vi "Create 256 Values Palette.vi"(5 "Image High Color":u32(colorbox), 7 "Image Low Color":u32(colorbox), 9 "Source Image Display Range":cluster{"Min Value":dbl, "Max Value":dbl}={"Min Value"=nan, "Max Value"=nan}, 10 "Interpolate?":bool, 11 "Palette Colors in":u32[](array[colorbox])) -> (0 "Color Scale Marker Values":T1(array[cluster]), 2 "1D U32 array":u32[](array[colorbox]), 3 "1D Color value array":cluster{"Red":u8, "Green":u8, "Blue":u8}[](array[cluster]))   [LabVIEW 2019]
uses:
  <vilib>/vision/NI_Vision_Development_Module.lvlib
panel:
  out "Color Ramp":dbl(ramp)
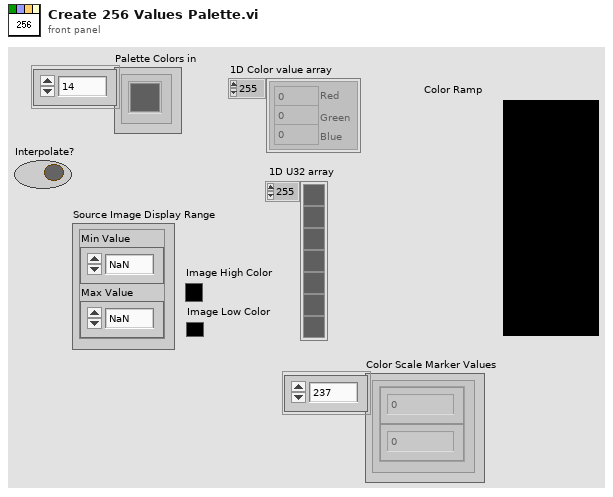
[diagram p1: front panel]
types:
  T1 = cluster{"Numeric Control":dbl, "Numeric Control":u32}[]
  T2 = typedef "For Loop Iteration Type.ctl" = enum16{"default", "first", "last", "out of range"}
  T3 = cluster{"Red (or Hue) value":u8, "Green (or Sat) value":u8, "Blue (or Light or Val) value":u8}[]
  T4 = cluster{"Red (or Hue) value":u8, "Green (or Sat) value":u8, "Blue (or Light or Val) value":u8}
  T5 = cluster{"Numeric Control":dbl, "Numeric Control":u32}
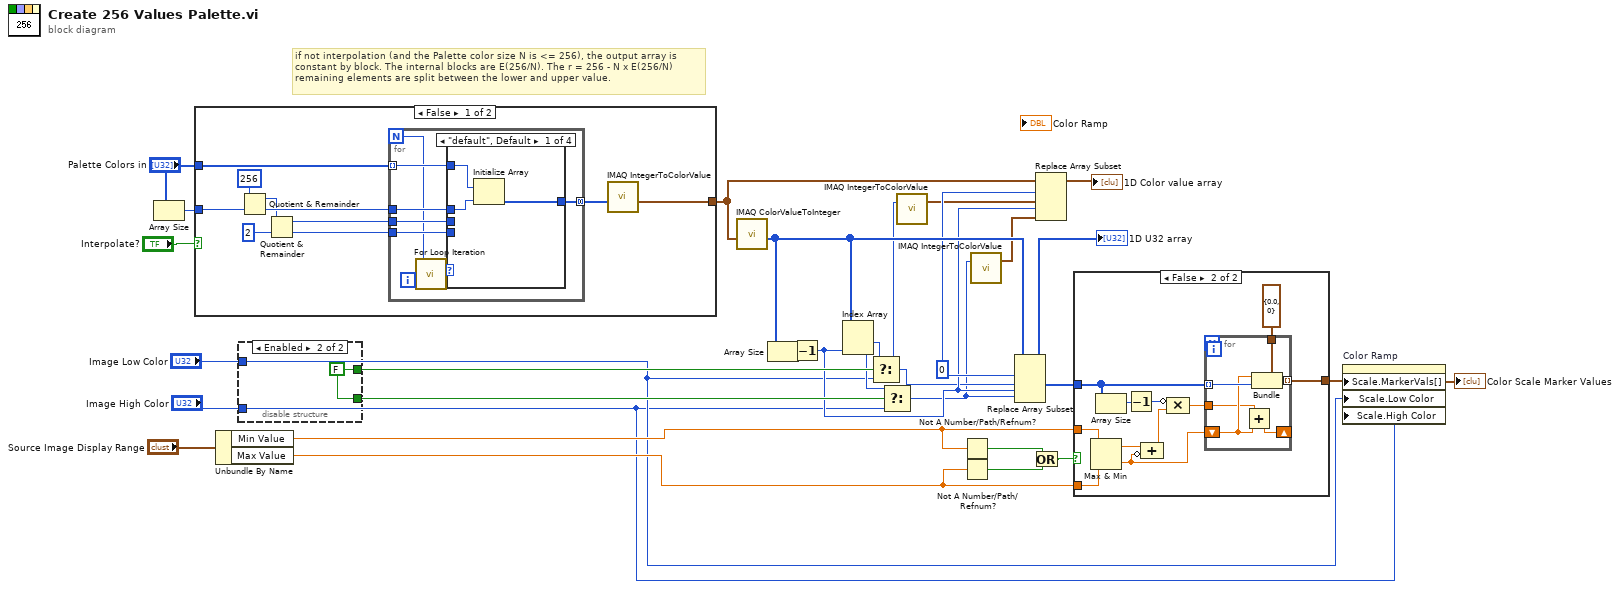
[diagram p0: block diagram]
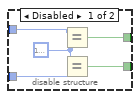
[diagram p2: hidden frame]
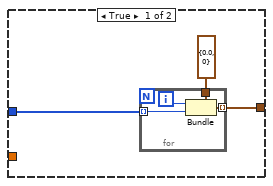
[diagram p3: hidden frame]
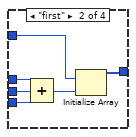
[diagram p4: hidden frame]
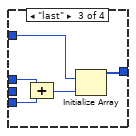
[diagram p5: hidden frame]
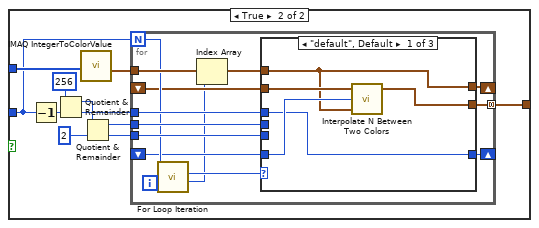
[diagram p7: hidden frame]
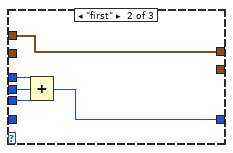
[diagram p8: hidden frame]
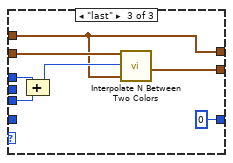
[diagram p9: hidden frame]
diagram:
  w9 = 0 ("index")
  # "if not interpolation (and the Palette color size N is <= 256), the output array is\nconstant by block. The internal blocks are E(256/N). The r = 256 - N x E(256/N)\nremaining elements are split between the lower and upper value."
  n1 = Array Size(array="Palette Colors in") -> (size(s)=w26:i32)
  n2 = case shown="False" "Interpolate?" {
    tunnel: w26 -> [w37 w61]
    tunnel: "Palette Colors in" -> [w32 w64]
    tunnel: [w28 w62] -> w10
    frame False {
      n3 = Quotient & Remainder(x=256, y=w37) -> (x-y*floor(x/y)=w35:i32, floor(x/y)=w36:i32)
      n4 = Quotient & Remainder(x=w35, y=2) -> (x-y*floor(x/y)=w33:i32, floor(x/y)=w31:i32)
      n5 = for {
        N -> [w38]
        tunnel: w36 -> [w43]
        tunnel: w31 -> [w45]
        tunnel: w33 -> [w44]
        tunnel: w32 -> [w41] mode=indexing
        tunnel: [w42] -> w29 mode=concatenating
        i -> [w40]
        n6 = call "For Loop Iteration.vi"("i"=w40, "N"=w38) -> ("Iteration"=w39:T2)  [unwired: 8 in, 1 out]
        n7 = case shown="\"default\", Default" w39 {
          tunnel: w45 -> [_ w54 w59 _]
          tunnel: w44 -> [_ w53 _ _]
          tunnel: w43 -> [w48 w52 w58 _]
          tunnel: w41 -> [w47 w50 w56 _]
          tunnel: [w46 w49 w55 _] -> w42
          frame "default", Default {
            n8 = Initialize Array(w47, w48) -> (w46:u32[])
          }
          frame "first" {
            n9 = Compound Arithmetic op=ADD(w52, w53, w54) -> (w51:i32)
            n10 = Initialize Array(w50, w51) -> (w49:u32[])
          }
          frame "last" {
            n11 = Compound Arithmetic op=ADD(w58, w59) -> (w57:i32)
            n12 = Initialize Array(w56, w57) -> (w55:u32[])
          }
          frame "out of range" {
          }
        }
      }
      n13 = call "IMAQ IntegerToColorValue"("1D U32 array"=w29) -> ("1D Color value array"=w28:T3)  [unwired: 4 in, 3 out]
    }
    frame True {
      n14 = Decrement(x=w61) -> (x-1=w60:i32)
      n15 = Quotient & Remainder(x=256, y=w60) -> (x-y*floor(x/y)=w69:i32, floor(x/y)=w70:i32)
      n16 = call "IMAQ IntegerToColorValue"("1D U32 array"=w64) -> ("1D Color value array"=w63:T3)  [unwired: 4 in, 3 out]
      n17 = Quotient & Remainder(x=w69, y=2) -> (x-y*floor(x/y)=w67:i32, floor(x/y)=w66:i32)
      n18 = for {
        N: w61 -> [w80]
        tunnel: w70 -> [w82]
        tunnel: w66 -> [w84]
        tunnel: w67 -> [w83]
        tunnel: w63 -> [w81]
        shift-right: [w77] -> _
        shift-left: _ -> [w75]
        shift-right: [w76] -> _
        shift-left: _ -> [w74]
        tunnel: [w73] -> w62 mode=concatenating
        i -> [w79]
        n19 = call "For Loop Iteration.vi"("i"=w79, "N"=w80) -> ("i (dup)"=w71:i32, "Iteration"=w78:T2)  [unwired: 8 in]
        n20 = Index Array(array=w81, index=w71) -> (element=w72:T4)
        n21 = case shown="\"default\", Default" w78 {
          tunnel: w84 -> [_ w94 w101]
          tunnel: w83 -> [_ w93 _]
          tunnel: w82 -> [w87 w92 w100]
          tunnel: w72 -> [w85 w91 w96]
          tunnel: [w85 w91 w96] -> w77
          tunnel: [w87 w90 0] -> w76
          tunnel: w75 -> [w86 _ w97]
          tunnel: w74 -> [w88 _ _]
          tunnel: [w89 _ w99] -> w73
          frame "default", Default {
            n22 = call "Interpolate N Between Two Colors.vi"("Starting Color Value"=w86, "# Elements"=w88, "Ending Color Value"=w85) -> ("Color Array"=w89:T3)  [unwired: 6 in]
          }
          frame "first" {
            n23 = Compound Arithmetic op=ADD(w92, w93, w94) -> (w90:i32)
          }
          frame "last" {
            n24 = Compound Arithmetic op=ADD(w100, w101) -> (w98:i32)
            n25 = call "Interpolate N Between Two Colors.vi"("Starting Color Value"=w97, "# Elements"=w98, "Ending Color Value"=w96) -> ("Color Array"=w99:T3)  [unwired: 6 in]
          }
        }
      }
    }
  }
  n26 = Unbundle By Name("Source Image Display Range") -> ("Min Value"=w21:dbl, "Max Value"=w20:dbl)
  n27 = disable-structure shown="Enabled" {
    disable-tunnel: [w105 w107] -> w17
    disable-tunnel: "Image Low Color" -> [w104 _]
    disable-tunnel: [w103 w107] -> w13
    disable-tunnel: "Image High Color" -> [w102 _]
    frame Disabled {
      w106 = u32 16777216 ("Image High Color")
      n28 = Equal?(x=w104, y=w106) -> (x = y?=w105:bool)
      n29 = Equal?(x=w106, y=w102) -> (x = y?=w103:bool)
    }
    frame Enabled {
      w107 = FALSE
    }
  }
  n30 = call "IMAQ ColorValueToInteger"("1D Color value array"=w10) -> ("1D U32 array"=w14:u32[])  [unwired: 4 in, 3 out]
  n31 = Array Size(array=w14) -> (size(s)=w15:i32)
  n32 = Decrement(x=w15) -> (x-1=w8:i32)
  n33 = Index Array(array=w14, index #2=w8) -> (element #1=w16:u32, element #2=w12:u32)  [unwired: 1 in]
  n34 = Select(t=w16, s=w17, f="Image Low Color") -> (s? t:f=w7:u32)
  n35 = Select(t=w12, s=w13, f="Image High Color") -> (s? t:f=w5:u32)
  n36 = call "IMAQ IntegerToColorValue"("U32 value"=w7) -> ("Color Value"=w6:T4)  [unwired: 4 in, 3 out]
  n37 = Not A Number/Path/Refnum?(number/path/refnum=w21) -> (NaN/Path/Refnum?=w24:bool)
  n38 = Not A Number/Path/Refnum?(number/path/refnum=w20) -> (NaN/Path/Refnum?=w23:bool)
  n39 = call "IMAQ IntegerToColorValue"("U32 value"=w5) -> ("Color Value"=w4:T4)  [unwired: 4 in, 3 out]
  n40 = Replace Array Subset(array=w14, new element #1=w7, index #1=w9, new element #2=w5, index #2=w8) -> (w11:u32[])
  "1D U32 array" <- w11
  n41 = Or(x=w24, y=w23) -> (x .or. y?=w18:bool)
  n42 = Replace Array Subset(array=w10, new element #1=w6, index #1=w9, new element #2=w4, index #2=w8) -> (→"1D Color value array":T3)
  n43 = case shown="False" w18 {
    tunnel: w11 -> [w110 w121]
    tunnel: [w109 w125] -> w19
    tunnel: w20 -> [_ w122]
    tunnel: w21 -> [_ w123]
    frame True {
      n44 = for {
        tunnel: w110 -> [w113] mode=indexing
        tunnel: [w112] -> w109 mode=indexing
        tunnel: T5 {"Numeric Control"=0.0, "Numeric Control"=0} ("Scale.Marker Values[]") -> [w111]
        i -> [w114]
        n45 = Bundle(cluster=w111, "Numeric Control"=w114, "Numeric Control"=w113) -> (w112:T5)
      }
    }
    frame False {
      n46 = Max & Min(x=w123, y=w122) -> (max(x,y)=w120:dbl, min(x,y)=w119:dbl)
      n47 = Array Size(array=w121) -> (size(s)=w118:i32)
      n48 = Decrement(x=w118) -> (x-1=w116:i32)
      n49 = Compound Arithmetic op=ADD(w120, invert w119) -> (w117:dbl)
      n50 = Compound Arithmetic op=MULTIPLY(invert w116, w117) -> (w115:dbl)
      n51 = for {
        tunnel: w121 -> [w131] mode=indexing
        tunnel: [w130] -> w125 mode=indexing
        tunnel: T5 {"Numeric Control"=0.0, "Numeric Control"=0} ("Scale.Marker Values[]") -> [w129]
        shift-right: [w126] -> _
        shift-left: w119 -> [w128]
        tunnel: w115 -> [w127]
        n52 = Add(x=w127, y=w128) -> (x+y=w126:dbl)
        n53 = Bundle(cluster=w129, "Numeric Control"=w128, "Numeric Control"=w131) -> (w130:T5)
      }
    }
  }
  "Color Scale Marker Values" <- w19
  n54 = property on="Color Ramp" class="ColRmp (strict)"("Scale.MarkerVals[]"=w19, "Scale.Low Color"="Image Low Color", "Scale.High Color"="Image High Color") -> ()  [unwired: 2 in, 2 out]
